vi "Tegam_Serial_Number.vi"(6 "simulation":string, 7 "Expected Model":string, 8 "Error In":errorcluster, 10 "Simulation":bool, 11 "GPIB Address":string="1") -> (0 "Error Out":errorcluster, 2 "Model":string, 3 "Serial Number":string)   [LabVIEW 2010]
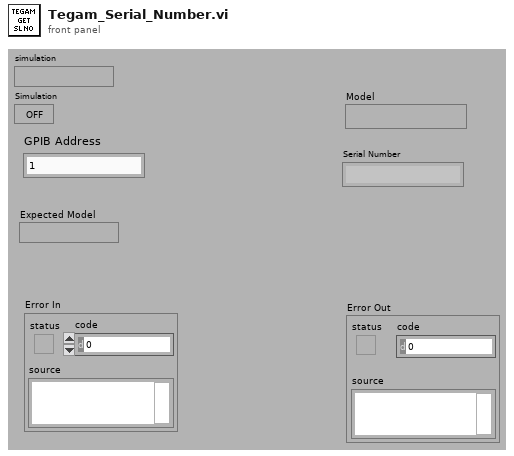
[diagram p1: front panel]
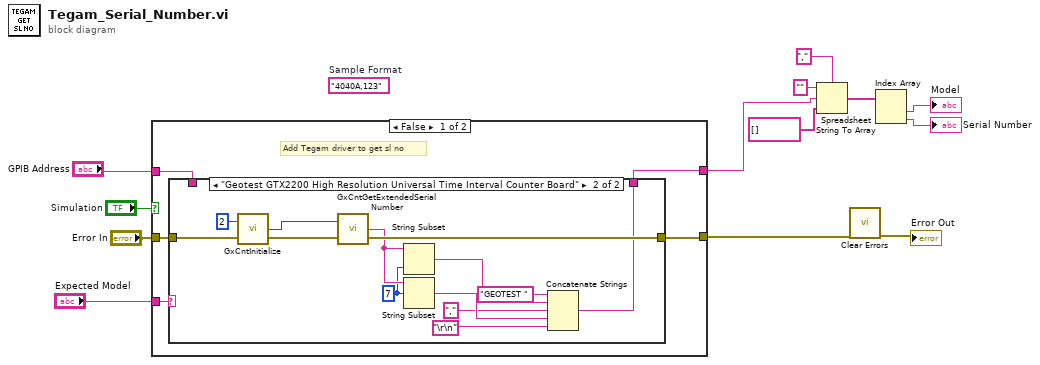
[diagram p0: block diagram]
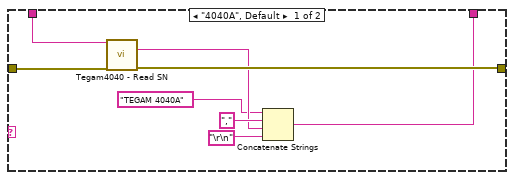
[diagram p2: hidden frame]
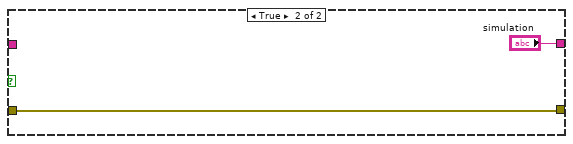
[diagram p3: hidden frame]
diagram:
  (unwired) "4040A,123"  # Sample Format
  n1 = case shown="False" "Simulation" {
    tunnel: "GPIB Address" -> [w15 _]
    tunnel: [w16 w41] -> w12
    tunnel: "Error In" -> [w17 w41]
    tunnel: [w14 "simulation"] -> w5
    tunnel: "Expected Model" -> [w18 _]
    frame False {
      # "Add Tegam driver to get sl no"
      n2 = case shown="\"Geotest GTX2200 High Resolution Universal Time Interval Counter Board\"" w18 {
        tunnel: w17 -> [w26 w39]
        tunnel: [w24 w37] -> w16
        tunnel: w15 -> [w25 _]
        tunnel: [w20 w31] -> w14
        frame "4040A", Default {
          n3 = call "Tegam4040 - Read SN.vi"("VISA TEGAM 4040A"=w25, "error in (no error)"=w26) -> ("Serial Number"=w21:string, "error out"=w24:errorcluster)  [unwired: 12 in]
          n4 = Concatenate Strings("TEGAM 4040A" ("string"), "," ("string"), w21, "\r\n") -> (w20:string)
        }
        frame "Geotest GTX2200 High Resolution Universal Time Interval Counter Board" {
          w29 = 7 ("offset (0)")
          n5 = call "GxCntInitialize.vi"("Slot"=i16 2, "error in (no error)"=w39) -> ("Handle"=w36:i16, "error out"=w38:errorcluster)  [unwired: 1 out]
          n6 = call "GxCntGetExtendedSerialNumber.vi"("Handle In"=w36, "error in (no error)"=w38) -> ("sSerialNumber"=w30:string, "error out"=w37:errorcluster)  [unwired: 1 out]
          n7 = String Subset(string=w30, length (rest)=w29) -> (substring=w28:string)  [unwired: 1 in]
          n8 = String Subset(string=w30, offset (0)=w29) -> (substring=w34:string)  [unwired: 1 in]
          n9 = Concatenate Strings("GEOTEST " ("string"), w28, "," ("string"), w34, "\r\n") -> (w31:string)
        }
      }
    }
    frame True {
    }
  }
  n10 = Spreadsheet String To Array(delimiter (Tab)=",", format string="", spreadsheet string=w5, array type (2D Dbl)=string[] []) -> (array=w6:string[])
  n11 = call <vilib>:"Clear Errors.vi"("error in (no error)"=w12) -> ("error out"=→"Error Out":errorcluster)  [unwired: 6 in]
  n12 = Index Array(array=w6) -> (element #1=→"Model":string, element #2=→"Serial Number":string)  [unwired: 2 in]
